vi "YAML.Scaler.vi"(2 "Key":string="Key", 3 "Scaler":string="Value") -> (1 "Output":string="Key: Value")   [LabVIEW 2016, in "Control Experiment.lvclass"]
uses:
  Control Experiment.lvclass
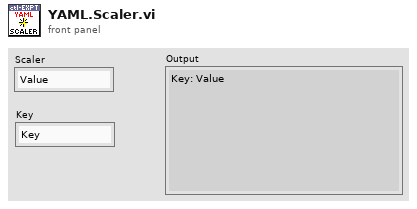
[diagram p1: front panel]
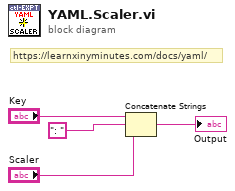
[diagram p0: block diagram]
diagram:
  # "https://learnxinyminutes.com/docs/yaml/"
  n1 = Concatenate Strings("Key", ": " ("string"), "Scaler") -> (→"Output":string)
